vi "Criteria Setting.vi"(8 "Error In":errorcluster, 11 "data in":string) -> (0 "Error Out":errorcluster, 2 "PASS?":string, 3 "Criteria":string)   [LabVIEW 2015]
panel:
  in  "Delete Button":bool
  in  "Save Button":bool
  in  "Lower Limit":string
  in  "Condition":enum16{"InBound", "OutBound"}(ring)
  in  "Upper Limit":string
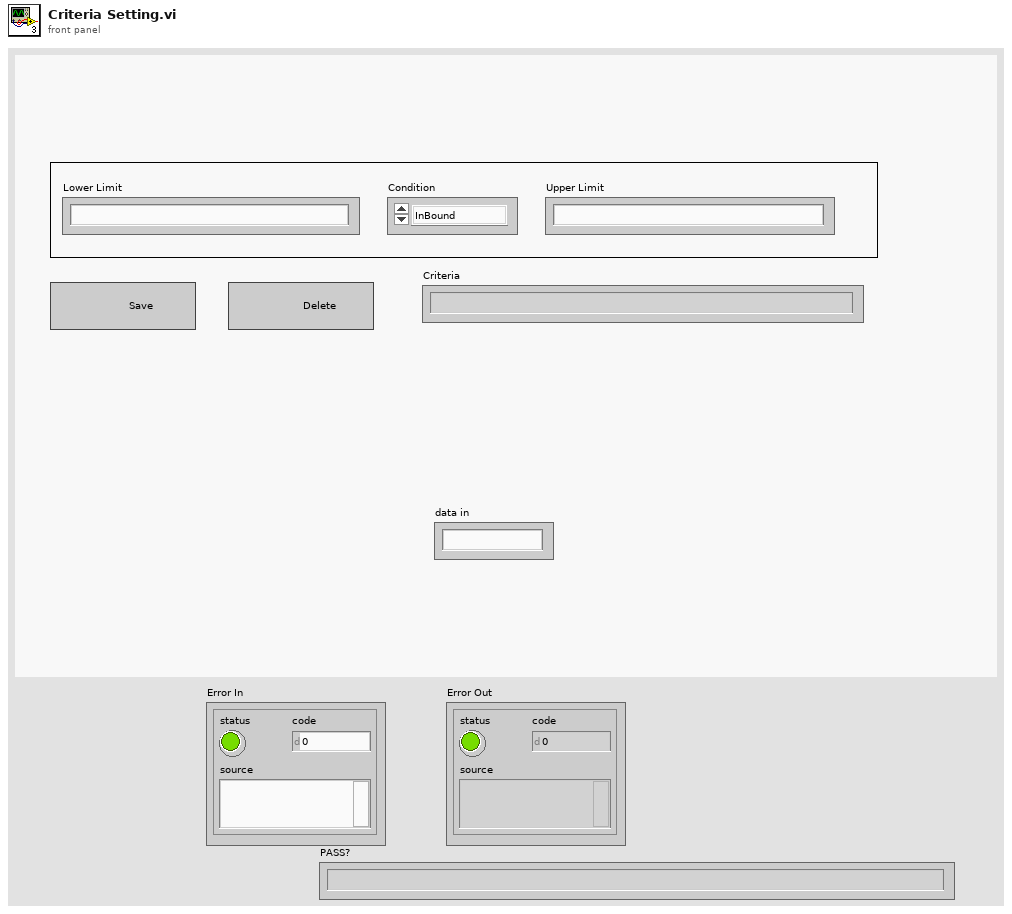
[diagram p1: front panel]
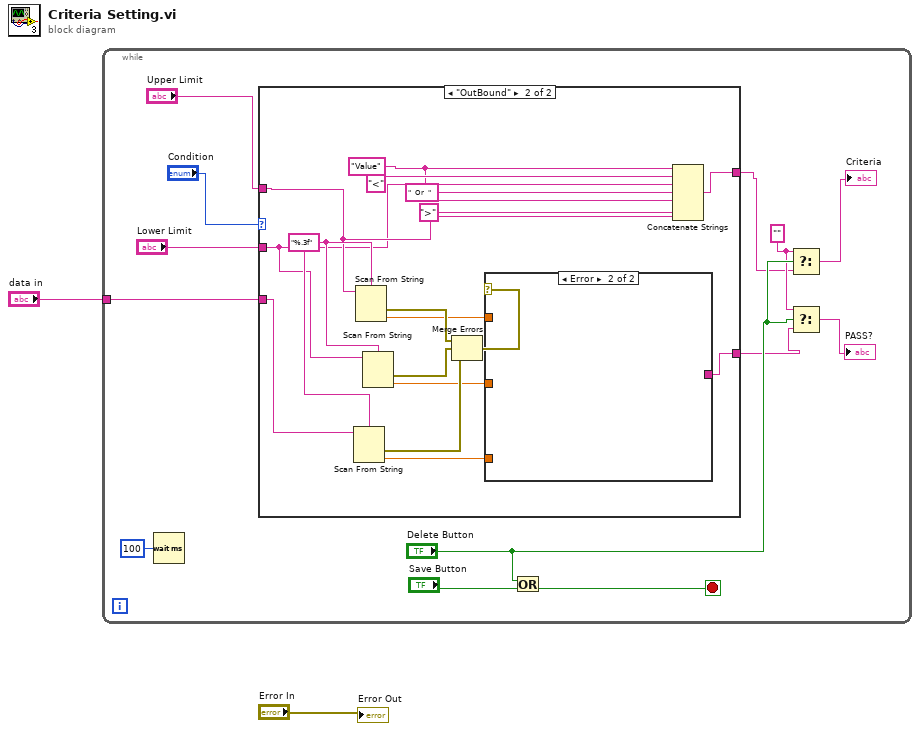
[diagram p0: block diagram]
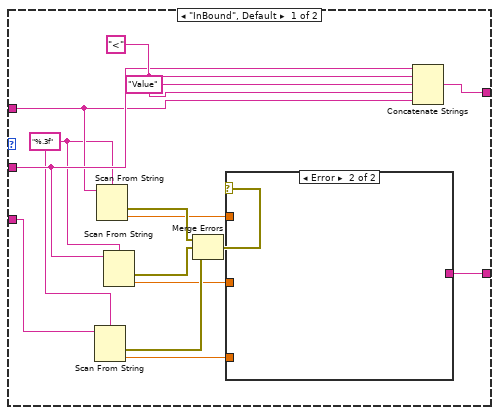
[diagram p2: hidden frame]
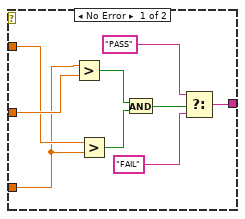
[diagram p3: hidden frame]
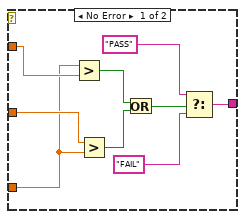
[diagram p4: hidden frame]
diagram:
  n1 = while {
    tunnel: "data in" -> [w10]
    stop <- w9 stop-if-true
    w7 = "" ("string")
    n2 = Wait (ms)(milliseconds to wait=u32 100) -> ()  [unwired: 1 out]
    n3 = case shown="\"OutBound\"" "Condition" {
      tunnel: "Lower Limit" -> [w27 w42]
      tunnel: "Upper Limit" -> [w25 w43]
      tunnel: [w29 w52] -> w6
      tunnel: w10 -> [w26 w41]
      tunnel: [w16 w40] -> w5
      frame "InBound", Default {
        w24 = "%.3f" ("format string")
        w30 = "<" ("string")
        n4 = Scan From String(format string=w24, input string=w26) -> (error out=w21:errorcluster, output 1=w19:dbl)  [unwired: 3 in, 2 out]
        n5 = Scan From String(format string=w24, input string=w25) -> (error out=w23:errorcluster, output 1=w17:dbl)  [unwired: 3 in, 2 out]
        n6 = Scan From String(format string=w24, input string=w27) -> (error out=w22:errorcluster, output 1=w18:dbl)  [unwired: 3 in, 2 out]
        n7 = Merge Errors(w23, w22, w21) -> (w20:errorcluster)
        n8 = case shown="Error" w20 {
          tunnel: w19 -> [w37 _]
          tunnel: w18 -> [w39 _]
          tunnel: w17 -> [w38 _]
          tunnel: [w31 _] -> w16
          frame No Error {
            n9 = Greater?(x=w37, y=w39) -> (0:w36:bool)
            n10 = Greater?(x=w38, y=w37) -> (0:w35:bool)
            n11 = And(x=w36, y=w35) -> (x .and. y?=w34:bool)
            n12 = Select(t="PASS" ("string"), s=w34, f="FAIL" ("string")) -> (s? t:f=w31:string)
          }
          frame Error {
          }
        }
        n13 = Concatenate Strings(w27, w30, "Value" ("string"), w30, w25) -> (w29:string)
      }
      frame "OutBound" {
        w51 = "%.3f" ("format string")
        w54 = "Value" ("string")
        n14 = Scan From String(format string=w51, input string=w41) -> (error out=w48:errorcluster, output 1=w46:dbl)  [unwired: 3 in, 2 out]
        n15 = Scan From String(format string=w51, input string=w43) -> (error out=w50:errorcluster, output 1=w44:dbl)  [unwired: 3 in, 2 out]
        n16 = Scan From String(format string=w51, input string=w42) -> (error out=w49:errorcluster, output 1=w45:dbl)  [unwired: 3 in, 2 out]
        n17 = Merge Errors(w50, w49, w48) -> (w47:errorcluster)
        n18 = case shown="Error" w47 {
          tunnel: w46 -> [w57 _]
          tunnel: w45 -> [w58 _]
          tunnel: w44 -> [w59 _]
          tunnel: [w60 _] -> w40
          frame No Error {
            n19 = Greater?(x=w57, y=w59) -> (0:w65:bool)
            n20 = Greater?(x=w58, y=w57) -> (0:w64:bool)
            n21 = Or(x=w65, y=w64) -> (x .or. y?=w63:bool)
            n22 = Select(t="PASS" ("string"), s=w63, f="FAIL" ("string")) -> (s? t:f=w60:string)
          }
          frame Error {
          }
        }
        n23 = Concatenate Strings(w54, "<" ("string"), w42, "  Or  " ("string"), w54, ">" ("string"), w43) -> (w52:string)
      }
    }
    n24 = Or(x="Delete Button", y="Save Button") -> (x .or. y?=w9:bool)
    n25 = Select(t=w7, s="Delete Button", f=w6) -> (s? t:f=→"Criteria":string)
    n26 = Select(t=w7, s="Delete Button", f=w5) -> (s? t:f=→"PASS?":string)
  }
  "Error Out" <- "Error In"
